vi "ILABW_ErrorToString.vi"(11 "errorIn":errorcluster) -> (3 "errorOut":string)   [LabVIEW 2012]
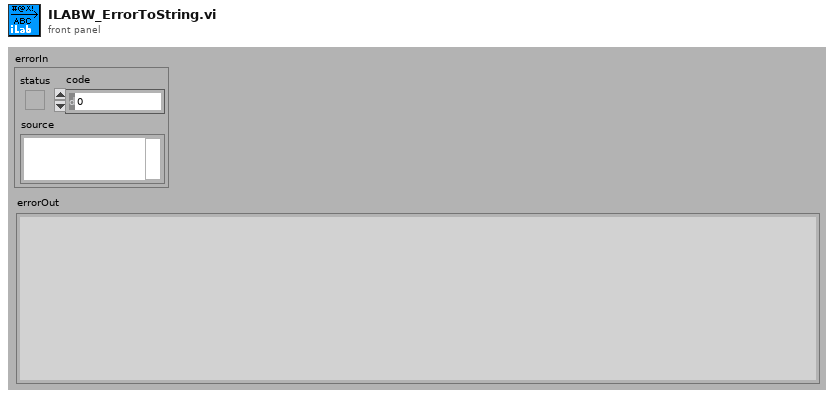
[diagram p1: front panel]
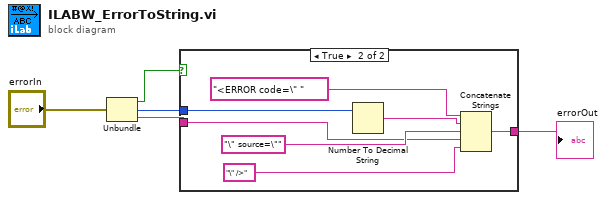
[diagram p0: block diagram]
diagram:
  n1 = Unbundle("errorIn") -> ("status"=w1:bool, "code"=w2:i32, "source"=w3:string)
  n2 = case shown="True" w1 {
    tunnel: [_ w8] -> w5
    tunnel: w3 -> [_ w7]
    tunnel: w2 -> [_ w6]
    frame False {
    }
    frame True {
      n3 = Number To Decimal String(number=w6) -> (decimal integer string=w9:string)  [unwired: 1 in]
      n4 = Concatenate Strings("<ERROR code=\" ", w9, "\" source=\"", w7, "\" />") -> (w8:string)
    }
  }
  "errorOut" <- w5
